vi "test string.vi"(8 "error in (no error)":errorcluster) -> (0 "error out":errorcluster)   [LabVIEW 2019, in "KH7008.lvlib"]
uses:
  KH7008.lvlib
  <vilib>/addons/_JKI Toolkits/Caraya/classes/Assert/Assert.lvclass
  <vilib>/addons/_JKI Toolkits/Caraya/classes/Test/Test.lvclass
  typedefs/filter--enum.ctl
  typedefs/couple--enum.ctl
  typedefs/shunt--enum.ctl
  typedefs/input--enum.ctl
  typedefs/gain--enum.ctl
  typedefs/channel--enum.ctl
  typedefs/channelProperties--Cluster.ctl
  <vilib>/addons/_JKI Toolkits/Caraya/classes/Assert/Assert Not Equal Value_Variant.vi
  <vilib>/addons/_JKI Toolkits/Caraya/classes/Assert/Assert Equal Value_Variant.vi
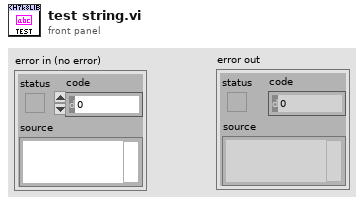
[diagram p1: front panel]
types:
  T1 = typedef "KH7008.lvlib/channelProperties--Cluster.ctl" = cluster{"Channel":T2, "Gain":T3, "Input Config":T4, "Shunt Resistor":T5, "Coupling":T6, "Bandwidth Filter":T7}
  T2 = typedef "KH7008.lvlib/channel--ring.ctl" = u32
  T3 = typedef "KH7008.lvlib/gain--Enum.ctl" = u8
  T4 = typedef "KH7008.lvlib/input--ring.ctl" = u16
  T5 = typedef "KH7008.lvlib/shunt--ring.ctl" = u32
  T6 = typedef "KH7008.lvlib/couple--enum.ctl" = enum16{"AC", "DC"}
  T7 = typedef "KH7008.lvlib/filter--enum.ctl" = enum16{"OFF", "ON"}
  T8 = cluster{"Channel":T2, "Gain":i32, "Input Config":i32, "Shunt Resistor":T5, "Coupling":i32, "Bandwidth Filter":i32}
  T9 = typedef "KH7008.lvlib/channelProperties--Cluster.ctl" = cluster{"channel":T10, "gain":T11, "input":T12, "shunt":T13, "couple":T6, "filter":T7}
  T10 = typedef "KH7008.lvlib/channel--enum.ctl" = enum16{"1", "2", "3", "4", "5", "6", "7", "8"}
  T11 = typedef "KH7008.lvlib/gain--enum.ctl" = enum16{"1x", "10x", "100x", "1000x"}
  T12 = typedef "KH7008.lvlib/input--enum.ctl" = enum16{"OFF", "SE+", "SE-", "DIFF"}
  T13 = typedef "KH7008.lvlib/shunt--enum.ctl" = enum16{"Open", "50", "500", "5k", "50k", "10M"}
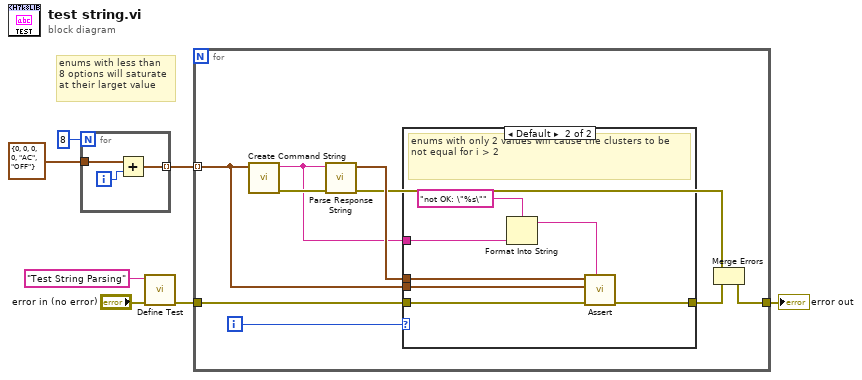
[diagram p0: block diagram]
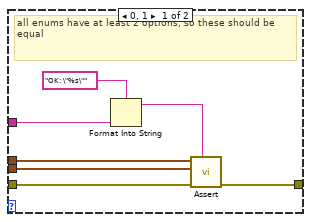
[diagram p2: hidden frame]
diagram:
  # "enums with less than\n8 options will saturate\nat their larget value"
  n1 = for {
    N: 8 -> [_]
    tunnel: T1 {"Channel"=0, "Gain"=0, "Input Config"=0, "Shunt Resistor"=0, "Coupling"=enum."AC", "Bandwidth Filter"=enum."OFF"} ("Channel Params") -> [w9]
    tunnel: [w8] -> w2 mode=indexing
    i -> [w10]
    n2 = Add(x=w9, y=w10) -> (x+y=w8:T8)
  }
  n3 = call <vilib>:"Define Test.vi"("error in (no error)"="error in (no error)", "Label (VI Title)"="Test String Parsing") -> ("error out"=w7:errorcluster)  [unwired: 8 in, 1 out]
  n4 = for {
    tunnel: w7 -> [w19]
    tunnel: [w12] -> w6
    tunnel: w2 -> [w17] mode=indexing
    i -> [w15]
    n5 = call "Create Command String.vi"("Channel Params"=w17) -> ("error out"=w18:errorcluster, "Command string"=w11:string)  [unwired: 9 in]
    n6 = call "Parse Response String.vi"("error in (no error)"=w18, "Response String"=w11) -> ("error out"=w14:errorcluster, "channelProperties"=w16:T9)  [unwired: 8 in]
    n7 = case shown="Default" w15 {
      tunnel: w19 -> [w26 w33]
      tunnel: [w25 w32] -> w13
      tunnel: w17 -> [w24 w31]
      tunnel: w16 -> [w23 w30]
      tunnel: w11 -> [w20 w28]
      frame 0, 1 {
        # "all enums have at least 2 options, so these should be equal"
        n8 = Format Into String(format string="OK: \"%s\"", w20) -> (resulting string=w22:string)  [unwired: 2 in, 1 out]
        n9 = call-poly <vilib>:"Assert.vi"("Label"=w22, "error in (no error)"=w26, "Y"=w24, "X"=w23) -> ("error out"=w25:errorcluster)  [unwired: 6 in, 1 out]
      }
      frame Default {
        # "enums with only 2 values will cause the clusters to be not equal for i > 2"
        n10 = Format Into String(format string="not OK: \"%s\"", w28) -> (resulting string=w27:string)  [unwired: 2 in, 1 out]
        n11 = call-poly <vilib>:"Assert.vi"("Label"=w27, "error in (no error)"=w33, "Y"=w31, "X"=w30) -> ("error out"=w32:errorcluster)  [unwired: 6 in, 1 out]
      }
    }
    n12 = Merge Errors(w14, w13) -> (w12:errorcluster)
  }
  "error out" <- w6
